vi "Build.vi"(0 "NI Build Specification_LV In":refnum<class "NI Build Specification_LV.lvclass">) -> (4 "NI Build Specification_LV Out":refnum<class "NI Build Specification_LV.lvclass">)   [LabVIEW 2017, in "CL_G3_VIComponentBuilder.lvlib" / "NI Build Specification_LV.lvclass"]
doc: "Creates the export artifacts, such as an executable, VI Package, DLL, etc."
uses:
  NI Build Specification_LV.lvclass
  C:/Tool Chain Support/Software Module Builder/Source/Exports/Exports/Export.lvclass
  Exports/Export.lvclass/Export.ctl
  Exports/Accessors/Read Export Build Specification.vi
  Exports/Accessors/Write Exported Build Specification Path.vi
  Exports/Accessors/Read Export Operation Errors.vi
  Exports/Accessors/Write Export Operation Errors.vi
  Exports/Export.lvclass
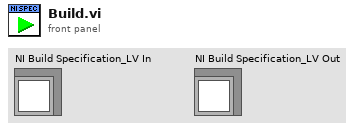
[diagram p1: front panel]
types:
  T1 = cluster{"Export":refnum<class "NI Build Specification_LV.lvclass">}
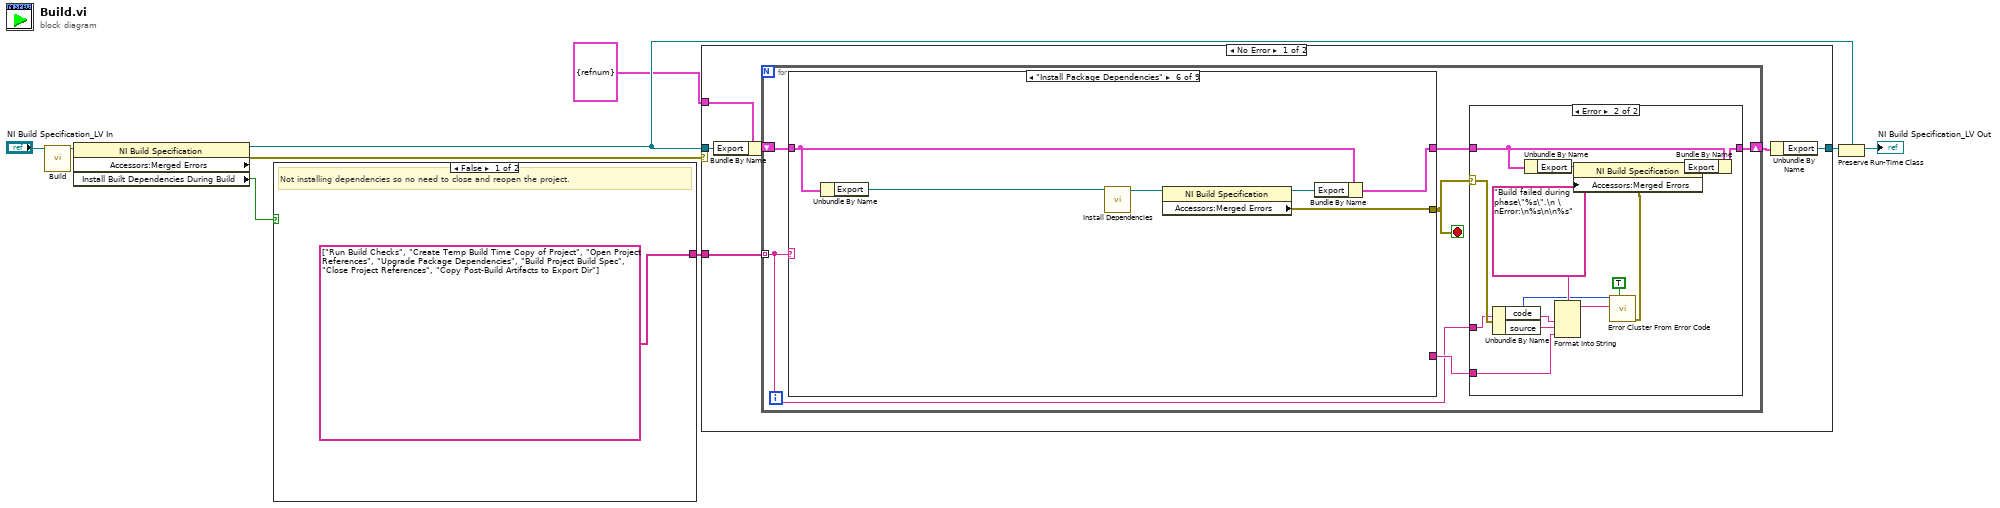
[diagram p0: block diagram]
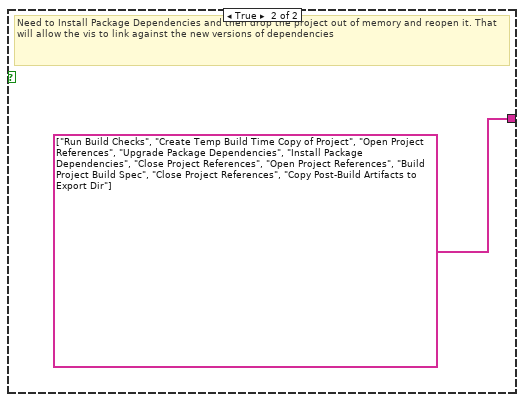
[diagram p2: hidden frame]
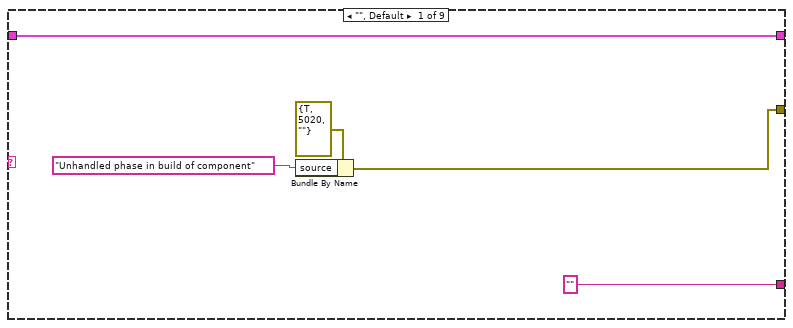
[diagram p3: hidden frame]
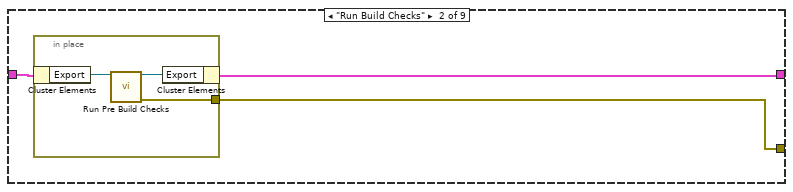
[diagram p4: hidden frame]
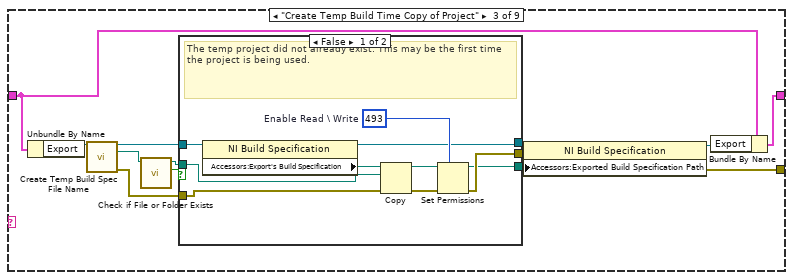
[diagram p5: hidden frame]
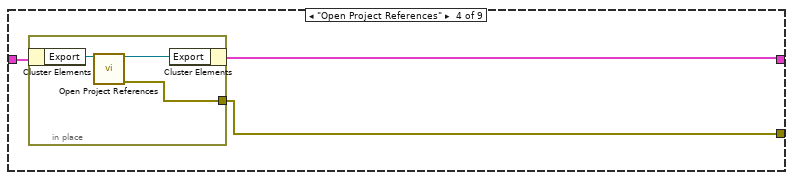
[diagram p7: hidden frame]
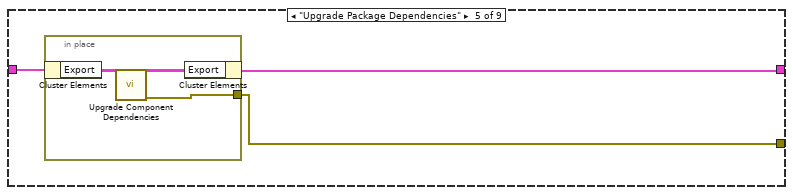
[diagram p8: hidden frame]
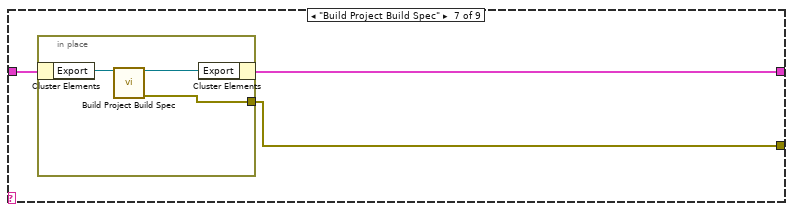
[diagram p9: hidden frame]
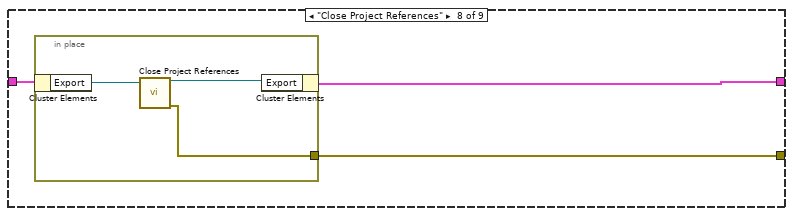
[diagram p10: hidden frame]
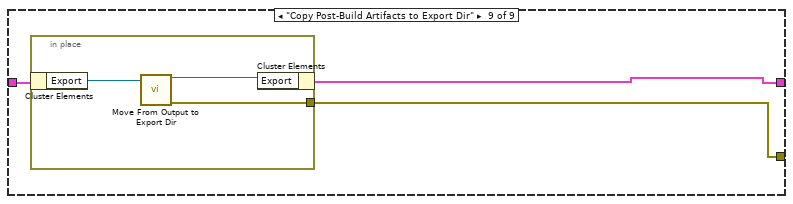
[diagram p11: hidden frame]
diagram:
  n1 = call-parent "Build.vi"("Export In"="NI Build Specification_LV In") -> ("Export Out"=w2:refnum<class "NI Build Specification_LV.lvclass">)  [unwired: 14 in]
  n2 = property class="NI Build Specification"(reference=w2) -> (reference out=w8:refnum<class "NI Build Specification_LV.lvclass">, "Accessors:Merged Errors"=w7:errorcluster, "Install Built Dependencies During Build"=w1:bool)  [unwired: 1 in, 1 out]
  n3 = case shown="False" w1 {
    tunnel: [string[] ["Run Build Checks", "Create Temp Build Time Copy of Project", "Open Project References", "Upgrade Package Dependencies", "Build Project Build Spec", "Close Project References", "Copy Post-Build Artifacts to Export Dir"] string[] ["Run Build Checks", "Create Temp Build Time Copy of Project", "Open Project References", "Upgrade Package Dependencies", "Install Package Dependencies", "Close Project References", "Open Project References", "Build Project Build Spec", "Close Project References", "Copy Post-Build Artifacts to Export Dir"]] -> w5
    frame False {
      # "Not installing dependencies so no need to close and reopen the project."
    }
    frame True {
      # "Need to Install Package Dependencies and then drop the project out of memory and reopen it. That will allow the vis to link against the new versions of dependencies"
    }
  }
  n4 = case shown="No Error" w7 {
    tunnel: w8 -> [w16 w111]
    tunnel: [w13 w111] -> w9
    tunnel: w5 -> [w17 _]
    tunnel: T1 {"Export"=refnum} -> [w12 _]
    frame No Error {
      n5 = Bundle By Name(cluster=w12, "Export"=w16) -> (w15:T1)
      n6 = for {
        shift-right: [w21] -> w14
        shift-left: w15 -> [w23]
        tunnel: w17 -> [w19] mode=indexing
        stop <- w18 stop-if-true
        n7 = case shown="\"Install Package Dependencies\"" w19 {
          tunnel: w23 -> [w28 w30 w47 w63 w69 w77 w81 w87 w93]
          tunnel: [w28 w29 w44 w62 w68 w76 w80 w86 w91] -> w22
          tunnel: [w26 w31 w39 w61 w67 w75 w79 w85 w92] -> w18
          tunnel: ["" ("format string") _ _ _ _ _ _ _ _] -> w20
          frame "", Default {
            n8 = Bundle By Name(cluster=errorcluster {"status"=TRUE, "code"=5020, "source"=""} ("error out"), "source"="Unhandled phase in build of component" ("format string")) -> (w26:errorcluster)
          }
          frame "Run Build Checks" {
            n9 = in-place {
              in-place-border: [w34] -> w31
              n10 = in-place-cluster #1(w30) -> ("Export"=w33:refnum<class "NI Build Specification_LV.lvclass">)
              n11 = call-dynamic "Run Pre Build Checks.vi"("NI Build Specification in"=w33) -> ("NI Build Specification out"=w32:refnum<class "NI Build Specification_LV.lvclass">, "error out"=w34:errorcluster)  [unwired: 13 in]
              n12 = in-place-cluster #1("Export"=w32) -> (w29:T1)
            }
          }
          frame "Create Temp Build Time Copy of Project" {
            n13 = Unbundle By Name(w47) -> ("Export"=w38:refnum<class "NI Build Specification_LV.lvclass">)
            n14 = call "Create Temp Build Spec File Name.vi"("Export"=w38) -> ("Export"=w37:refnum<class "NI Build Specification_LV.lvclass">, "Temporary build spec Path"=w36:path, "error IO"=w35:errorcluster)  [unwired: 12 in]
            n15 = call <vilib>:"Check if File or Folder Exists.vi"("path"=w36) -> ("file or folder exists?"=w45:bool, "dup path"=w46:path)  [unwired: 8 in, 1 out]
            n16 = case shown="False" w45 {
              tunnel: w37 -> [w56 w59]
              tunnel: w46 -> [w55 w60]
              tunnel: [w51 w59] -> w43
              tunnel: [w50 w58] -> w42
              tunnel: [w49 w60] -> w41
              tunnel: w35 -> [w48 w58]
              frame False {
                w52 = i16 493  # Enable Read \ Write
                # "The temp project did not already exist. This may be the first time the project is being used."
                n17 = property class="NI Build Specification"(reference=w56) -> (reference out=w51:refnum<class "NI Build Specification_LV.lvclass">, "Accessors:Export's Build Specification"=w57:path)  [unwired: 1 in, 1 out]
                n18 = Copy(8:w48, 10:w55, 11:w57) -> (0:w53:errorcluster, 3:w54:path)  [unwired: 2 in, 1 out]
                n19 = Set Permissions(7:w52, 8:w53, 11:w54) -> (0:w50:errorcluster, 3:w49:path)  [unwired: 2 in]
              }
              frame True {
                # "The temp project already exsists. This may happen because it is possible to define multiple build specifications same project and build more than one of those build specifications during the same build session."
              }
            }
            n20 = property class="NI Build Specification"(reference=w43, error in=w42, "Accessors:Exported Build Specification Path"=w41) -> (reference out=w40:refnum<class "NI Build Specification_LV.lvclass">, error out=w39:errorcluster)
            n21 = Bundle By Name(cluster=w47, "Export"=w40) -> (w44:T1)
          }
          frame "Open Project References" {
            n22 = in-place {
              in-place-border: [w64] -> w61
              n23 = in-place-cluster #2(w63) -> ("Export"=w66:refnum<class "NI Build Specification_LV.lvclass">)
              n24 = call-dynamic "Open Project References.vi"("NI Build Specification"=w66) -> ("NI Build Specification"=w65:refnum<class "NI Build Specification_LV.lvclass">, "error out"=w64:errorcluster)  [unwired: 13 in]
              n25 = in-place-cluster #2("Export"=w65) -> (w62:T1)
            }
          }
          frame "Upgrade Package Dependencies" {
            n26 = in-place {
              in-place-border: [w72] -> w67
              n27 = in-place-cluster #3(w69) -> ("Export"=w71:refnum<class "NI Build Specification_LV.lvclass">)
              n28 = call-dynamic "Upgrade Component Dependencies.vi"("NI Build Specification_LV In"=w71) -> ("NI Build Specification_LV Out"=w70:refnum<class "NI Build Specification_LV.lvclass">, "error out"=w72:errorcluster)  [unwired: 13 in]
              n29 = in-place-cluster #3("Export"=w70) -> (w68:T1)
            }
          }
          frame "Install Package Dependencies" {
            n30 = Unbundle By Name(w77) -> ("Export"=w78:refnum<class "NI Build Specification_LV.lvclass">)
            n31 = call-dynamic "Install Dependencies.vi"("Export in"=w78) -> ("Export out"=w74:refnum<class "NI Build Specification_LV.lvclass">)  [unwired: 14 in]
            n32 = property class="NI Build Specification"(reference=w74) -> (reference out=w73:refnum<class "NI Build Specification_LV.lvclass">, "Accessors:Merged Errors"=w75:errorcluster)  [unwired: 1 in, 1 out]
            n33 = Bundle By Name(cluster=w77, "Export"=w73) -> (w76:T1)
          }
          frame "Build Project Build Spec" {
            n34 = in-place {
              in-place-border: [w82] -> w79
              n35 = in-place-cluster #4(w81) -> ("Export"=w84:refnum<class "NI Build Specification_LV.lvclass">)
              n36 = call-dynamic "Build Project Build Spec.vi"("NI Build Specification in"=w84) -> ("NI Build Specification out"=w83:refnum<class "NI Build Specification_LV.lvclass">, "error out"=w82:errorcluster)  [unwired: 13 in]
              n37 = in-place-cluster #4("Export"=w83) -> (w80:T1)
            }
          }
          frame "Close Project References" {
            n38 = in-place {
              in-place-border: [w88] -> w85
              n39 = in-place-cluster #5(w87) -> ("Export"=w90:refnum<class "NI Build Specification_LV.lvclass">)
              n40 = call-dynamic "Close Project References.vi"("NI Build Specification in"=w90) -> ("NI Build Specification out"=w89:refnum<class "NI Build Specification_LV.lvclass">, "error out"=w88:errorcluster)  [unwired: 13 in]
              n41 = in-place-cluster #5("Export"=w89) -> (w86:T1)
            }
          }
          frame "Copy Post-Build Artifacts to Export Dir" {
            n42 = in-place {
              in-place-border: [w94] -> w92
              n43 = in-place-cluster #6(w93) -> ("Export"=w96:refnum<class "NI Build Specification_LV.lvclass">)
              n44 = call-dynamic "Move From Output to Export Dir.vi"("NI Build Specification in"=w96) -> ("NI Build Specification out"=w95:refnum<class "NI Build Specification_LV.lvclass">, "error out"=w94:errorcluster)  [unwired: 13 in]
              n45 = in-place-cluster #6("Export"=w95) -> (w91:T1)
            }
          }
        }
        n46 = case shown="Error" w18 {
          selector: w18 -> [_ w108]
          tunnel: [w97 w106] -> w21
          tunnel: w22 -> [w97 w107]
          tunnel: w20 -> [_ w101]
          tunnel: w19 -> [_ w99]
          frame No Error {
          }
          frame Error {
            n47 = Unbundle By Name(w108) -> ("code"=w98:i32, "source"=w100:string)
            n48 = Unbundle By Name(w107) -> ("Export"=w105:refnum<class "NI Build Specification_LV.lvclass">)
            n49 = Format Into String(format string="Build failed during phase\"%s\".\n \nError:\n%s\n\n%s" ("error message (\"\")"), w99, w100, w101) -> (resulting string=w109:string)  [unwired: 2 in, 1 out]
            n50 = call <vilib>:"Error Cluster From Error Code.vi"("show call chain? (False)"=TRUE, "error message (\"\")"=w109, "error code (0)"=w98) -> ("error out"=w103:errorcluster)  [unwired: 6 in]
            n51 = property class="NI Build Specification"(reference=w105, "Accessors:Merged Errors"=w103) -> (reference out=w104:refnum<class "NI Build Specification_LV.lvclass">)  [unwired: 1 in, 1 out]
            n52 = Bundle By Name(cluster=w107, "Export"=w104) -> (w106:T1)
          }
        }
      }
      n53 = Unbundle By Name(w14) -> ("Export"=w13:refnum<class "NI Build Specification_LV.lvclass">)
    }
    frame Error {
    }
  }
  n54 = Preserve Run-Time Class(object in=w9, 2:w8) -> (object out=→"NI Build Specification_LV Out":refnum<class "NI Build Specification_LV.lvclass">)  [unwired: 1 in, 1 out]
